vi "file.Read.vi"(8 "error in":errorcluster, 11 "Folder":path) -> (0 "error out":errorcluster, 2 "enabled":bool, 3 "u16 pixmap":T1)   [LabVIEW 2020]
uses:
  _controls/img.u16.graph.25pc.axes.ctl
  <vilib>/Utility/miscctls.llb/LVPointTypeDef.ctl
  cc16ed15-0944-4734-9224-23c8f639c3b2.vi
  file.IsValid.vi
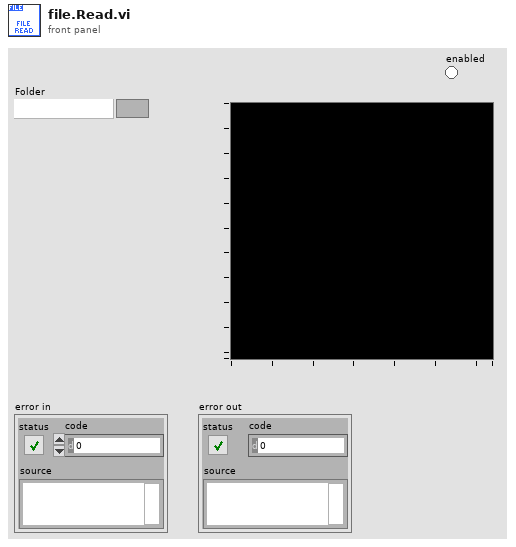
[diagram p1: front panel]
types:
  T1 = typedef "img.u16.graph.25pc.axes.ctl" = u16[][]
  T2 = typedef "LVPointTypeDef.ctl" = cluster{"Horizontal":i16, "Vertical":i16}
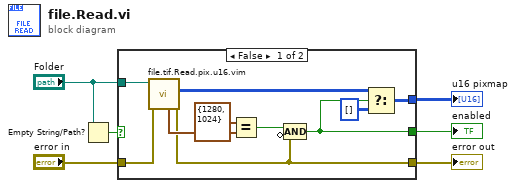
[diagram p0: block diagram]
diagram:
  n1 = Empty String/Path?(string/path="Folder") -> (empty?=w2:bool)
  n2 = case shown="False" w2 {
    tunnel: "Folder" -> [w16 _]
    tunnel: "error in" -> [w15 w17]
    tunnel: [w7 w17] -> w4
    tunnel: [w12 _] -> w3
    tunnel: [w9 _] -> w6
    frame False {
      n3 = call "file.tif.Read.pix.u16.vim"("error in"=w15, "path"=w16) -> ("error out"=w7:errorcluster, "u16 pixmap"=w10:T1, "size"=w8:T2)  [unwired: 5 in, 2 out]
      n4 = Equal?(x=T2 {"Horizontal"=1280, "Vertical"=1024} ("size 2"), y=w8) -> (x = y?=w13:bool)
      n5 = Compound Arithmetic op=AND(w13, invert w7) -> (w12:bool)
      n6 = Select(t=w10, s=w12, f=T1 []) -> (s? t:f=w9:T1)
    }
    frame True {
    }
  }
  "u16 pixmap" <- w6
  "error out" <- w4
  "enabled" <- w3
